vi "Main UI.vi"() -> ()   [LabVIEW 2013]
uses:
  Refactor/TypeDefs/Throttle.ctl
  Refactor/TypeDefs/Steering.ctl
  <vilib>/userdefined/High Color/IMAQdx.ctl
  Refactor/TypeDefs/PhoneIMU.ctl
  <vilib>/Utility/inputDevices.llb/joystickAcquire.vi
  PCTx Files/PCTx/PCTx.lvlib
  <vilib>/vision/driver/NI_Vision_Acquisition_Software.lvlib
  <resource>/objmgr/imaqdx.rc
  FFConstdll/FFConstDll.dll
  user32.dll
panel:
  out "Gear":i32
  in  "Tab Control":enum32{"HUD", "Stats for Nerds", "Debug Info"}(tab)
  in  "stop":bool
  out "Steering":i32(knob) scale=-32768.0..32767.0
  out "Throttle":i32(knob) scale=-32768.0..32767.0
  out "Brake":i32(slide) scale=32767.0..-32768.0
  out "Image":T1(plugin-control)
  out "Throttle Graph":cluster{dbl[], dbl[]}[](graph)
  out "Steering Graph":cluster{dbl[], dbl[]}[](graph)
  out "Raw Wheel Inputs":T2
  in  "Throttle Cluster":T3={"Neutral Signal"=512.0, "Bottom Deadzone"=707.070707070707, "Neutral Deadzone"=0.0, "Top Cutout"=971.4285714285714, "Bottom Cutout"=89.79591836734694, "Top Deadzone"=64627.90909090909, "Throttle Curve Type"=enum."Linear"} {"Top Deadzone" scale=55537.0..65537.0; "Bottom Cutout" scale=0.0..200.0; "Top Cutout" scale=800.0..1024.0; "Neutral Deadzone" scale=0.0..10000.0; "Bottom Deadzone" scale=1.0..10000.0; "Neutral Signal" scale=480.0..544.0}
  in  "Steering Cluster":T4={"Neutral Signal"=642.8571428571429, "Bottom Deadzone"=707.070707070707, "Neutral Deadzone"=0.0, "Top Cutout"=971.4285714285714, "Bottom Cutout"=89.79591836734694, "Top Deadzone"=64627.90909090909, "Throttle Curve Type"=enum."Linear"} {"Top Deadzone" scale=32768.0..65537.0; "Bottom Cutout" scale=0.0..512.0; "Top Cutout" scale=800.0..1024.0; "Neutral Deadzone" scale=0.0..10000.0; "Bottom Deadzone" scale=1.0..32767.0; "Neutral Signal" scale=420.0..700.0}
  out "Steering PPM":dbl
  out "Throttle PPM":dbl
  in  "Min Throttle":dbl=513.0
  in  "Min Reverse":dbl=511.0
  in  "CD timer":u32=250
  in  "Camera Name":T5="cam0"
  in  "Video Modes":i32(listbox)=22
  out "Start ForegroundWindow HWND":u32
  in  "nXForce":i32(slide) scale=-10000.0..10000.0
  out "SetDeviceForce HRESULT":i32
  out "Acquire HRESULT":i32
  out "Current ForegroundWindow HWND":u32
  in  "millisecond multiple":u32=50
  out "Init HRESULT":i32
  out "button info":T6
  in  "Host Port":u16=55555
  out "Source Address":u32
  out "Time Since Last Packet":u32
  out "Iteration":i32
  out "Length":i32
  out "Source Port":u16
  out "data out":string
  out "IMU Data Array":dbl[](array[numeric])
  out "output cluster":T7
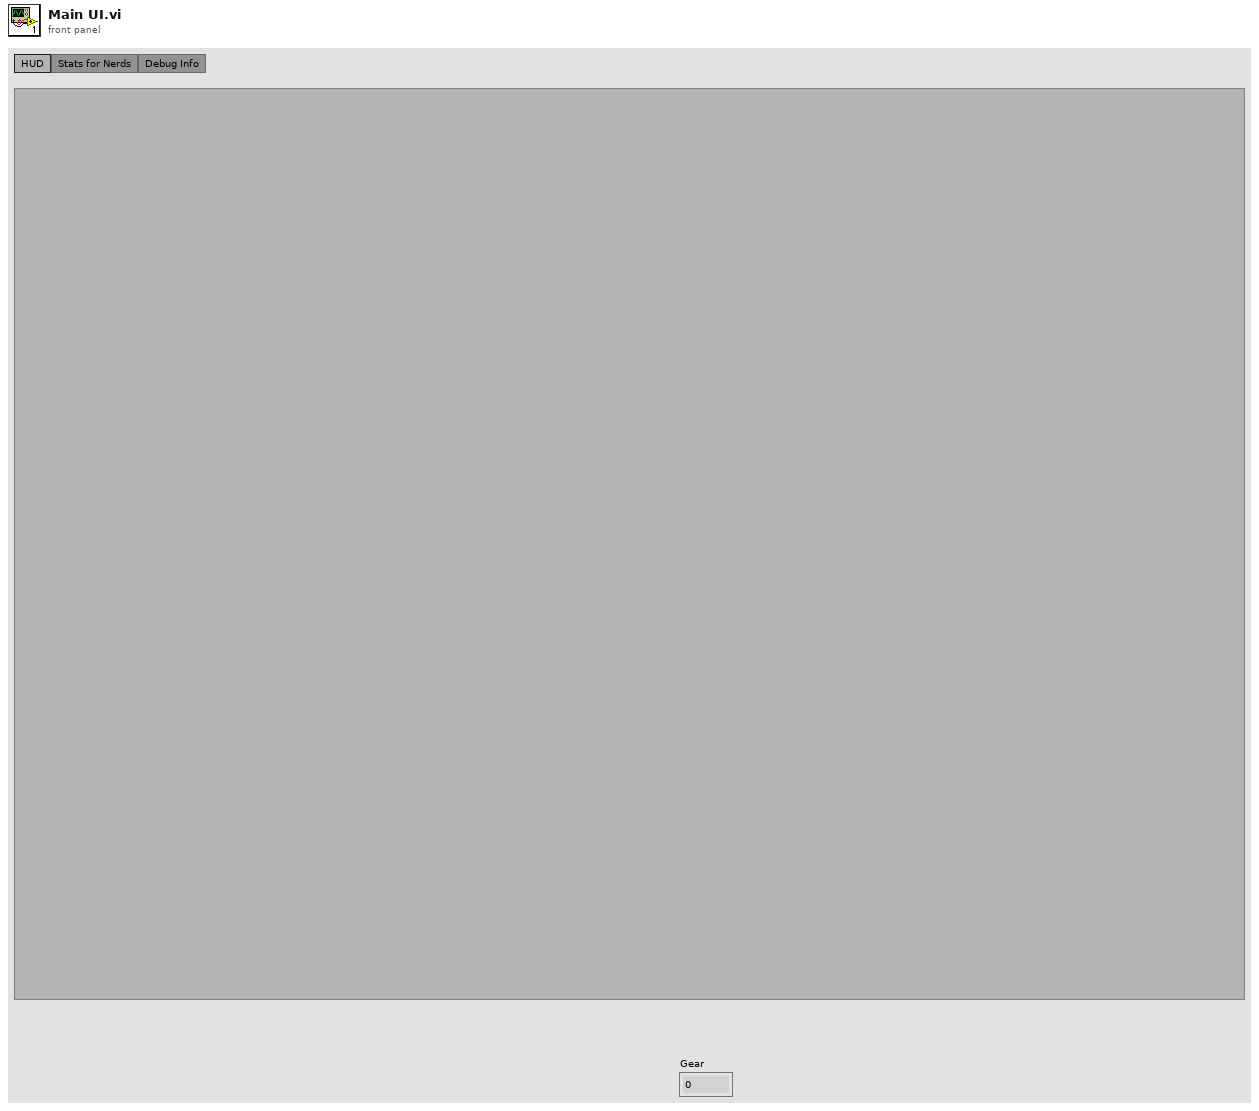
[diagram p1: front panel]
types:
  T1 = typedef "IMAQ Image.ctl" = refnum<image>
  T2 = cluster{"X axis":i32, "Y axis":i32, "Z axis":i32, "X axis rotation":i32, "Y axis rotation":i32, "Z axis rotation":i32, "U axis":i32, "V axis":i32}
  T3 = typedef "Throttle.ctl" = cluster{"Neutral Signal":dbl, "Bottom Deadzone":dbl, "Neutral Deadzone":dbl, "Top Cutout":dbl, "Bottom Cutout":dbl, "Top Deadzone":dbl, "Throttle Curve Type":enum16{"Linear", "Linear, No Deadzone", "Logarithmic", "Exponental"}}
  T4 = typedef "Steering.ctl" = cluster{"Neutral Signal":dbl, "Bottom Deadzone":dbl, "Neutral Deadzone":dbl, "Top Cutout":dbl, "Bottom Cutout":dbl, "Top Deadzone":dbl, "Throttle Curve Type":enum16{"Linear", "Linear, No Deadzone", "Logarithmic", "Exponental"}}
  T5 = typedef "IMAQdx.ctl" = refnum<k21>
  T6 = cluster{"X":bool, "Square":bool, "Circle":bool, "Triangle":bool, "Right Paddle":bool, "Left Paddle":bool, "R2":bool, "L2":bool, "Select":bool, "Start":bool, "R3":bool, "L3":bool, "Shifter +":bool, "Shifter -":bool, "Enter":bool, "Plus":bool, "Ring Clockwise":bool, "Ring CCW":bool, "Minus":bool, "GT (Center)":bool, "PS":bool, "button 22":bool, "button 23":bool, "button 24":bool, "button 25":bool, "button 26":bool, "button 27":bool, "button 28":bool, "button 29":bool, "button 30":bool, "button 31":bool, "button 32":bool}
  T7 = cluster{"Z Gyroscope":dbl, "Y Accelerometer":dbl, "X Gyroscope":dbl, "Timestamp":dbl, "Y Gyroscope":dbl, "Z Accelerometer":dbl, "GPS 5":dbl, "X Accelerometer":dbl, "X Magnetic Field":dbl, "Y Magnetic Field":dbl, "Z Magnetic Field":dbl, "GPS 1":dbl, "GPS 2":dbl, "GPS 3":dbl, "GPS 4":dbl, "GPS 6":dbl}
  T8 = typedef "PhoneIMU.ctl" = cluster{"Z Gyroscope":dbl, "Y Accelerometer":dbl, "X Gyroscope":dbl, "Timestamp":dbl, "Y Gyroscope":dbl, "Z Accelerometer":dbl, "GPS 5":dbl, "X Accelerometer":dbl, "X Magnetic Field":dbl, "Y Magnetic Field":dbl, "Z Magnetic Field":dbl, "GPS 1":dbl, "GPS 2":dbl, "GPS 3":dbl, "GPS 4":dbl, "GPS 6":dbl}
  T9 = typedef "Image Type" = u32
  T10 = cluster{"button 1":bool, "button 2":bool, "button 3":bool, "button 4":bool, "button 5":bool, "button 6":bool, "button 7":bool, "button 8":bool, "button 9":bool, "button 10":bool, "button 11":bool, "button 12":bool, "button 13":bool, "button 14":bool, "button 15":bool, "button 16":bool, "button 17":bool, "button 18":bool, "button 19":bool, "button 20":bool, "button 21":bool, "button 22":bool, "button 23":bool, "button 24":bool, "button 25":bool, "button 26":bool, "button 27":bool, "button 28":bool, "button 29":bool, "button 30":bool, "button 31":bool, "button 32":bool}
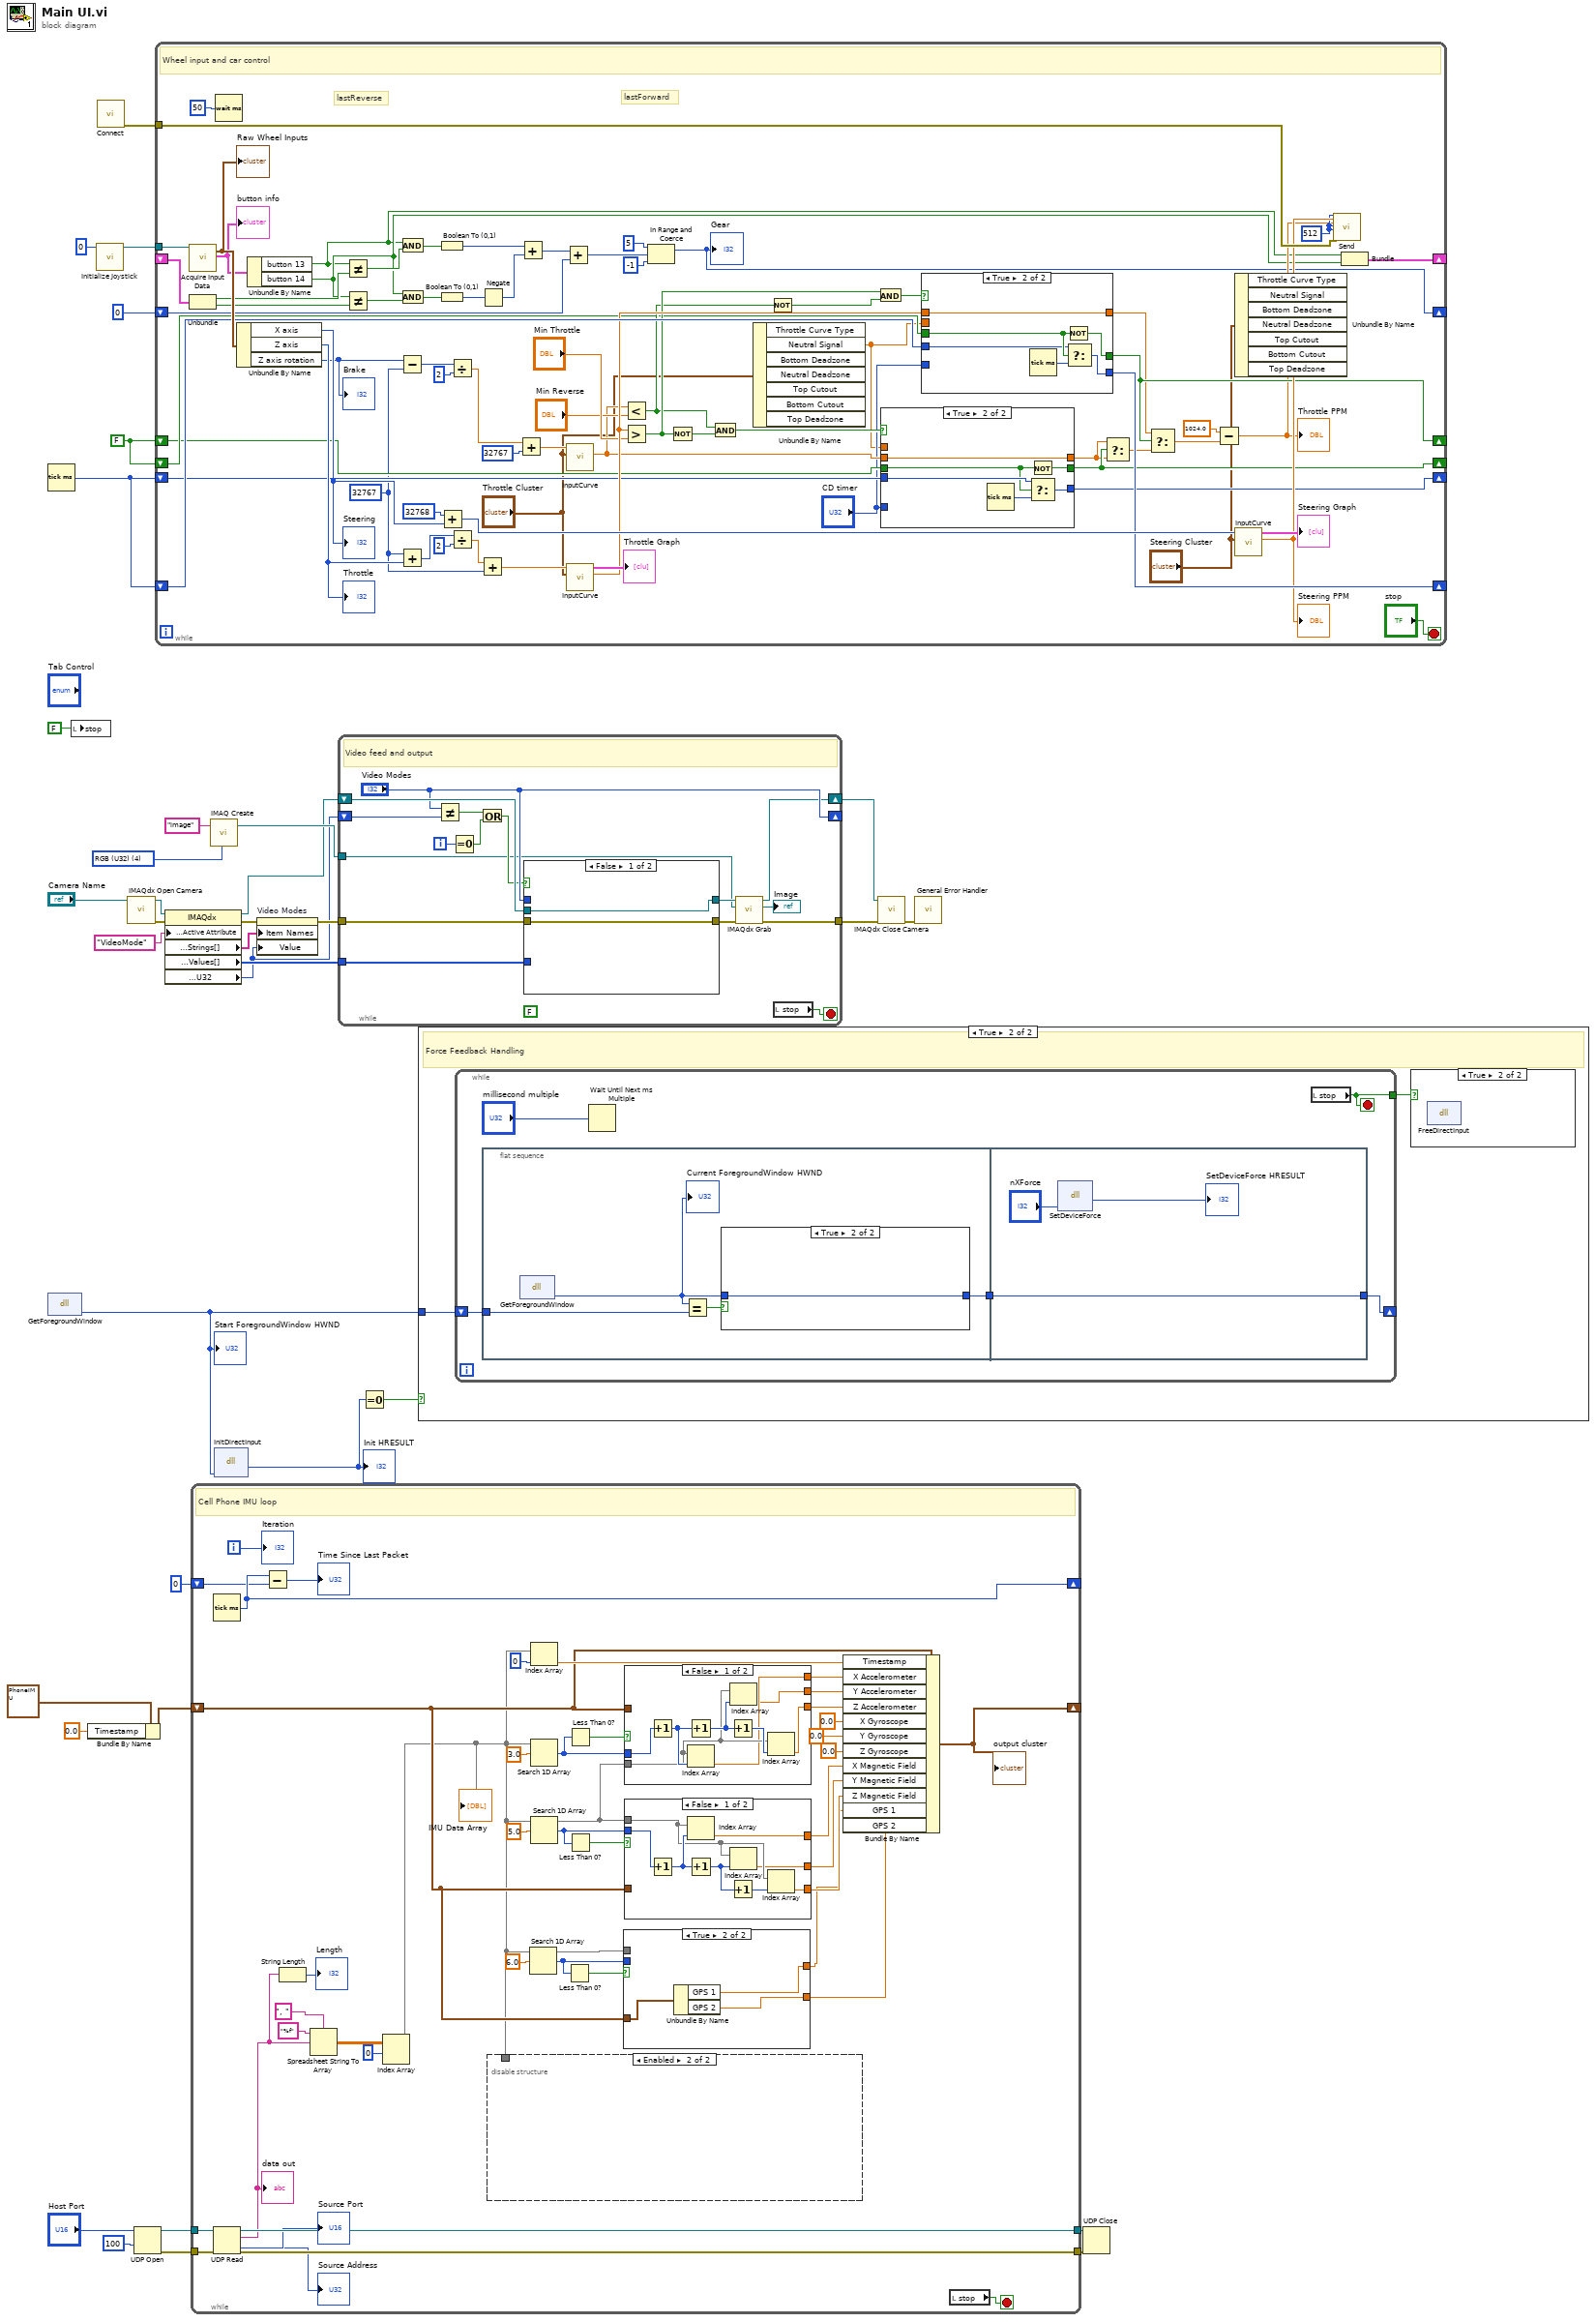
[diagram p0: block diagram]
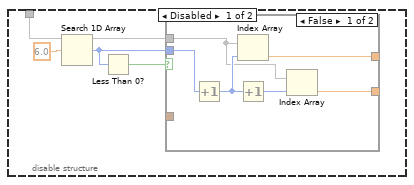
[diagram p2: hidden frame]
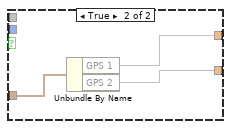
[diagram p3: hidden frame]
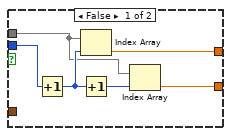
[diagram p4: hidden frame]
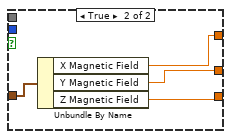
[diagram p5: hidden frame]
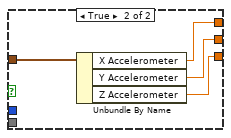
[diagram p6: hidden frame]
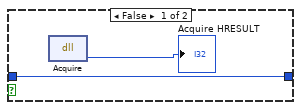
[diagram p9: hidden frame]
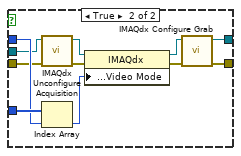
[diagram p10: hidden frame]
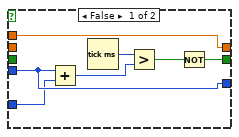
[diagram p11: hidden frame]
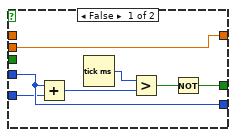
[diagram p12: hidden frame]
diagram:
  w16 = T9 4 items=["Grayscale (U8)", "Grayscale (I16)", "Grayscale (SGL)", "Complex (CSG)", "RGB (U32)", "HSL (U32)", "RGB (U64)", "Grayscale (U16)"] ("Image Type")
  w32 = FALSE
  n1 = Tick Count (ms)() -> (millisecond timer value=w33:u32)
  n2 = dll-call lib="user32.dll" fn="GetForegroundWindow"() -> ("HWND"=w13:u32)  [unwired: 3 in, 2 out]
  "Start ForegroundWindow HWND" <- w13
  n3 = local write "stop"(FALSE ("stop")) -> ()
  n4 = Bundle By Name(cluster=T8 {"Z Gyroscope"=0.0, "Y Accelerometer"=0.0, "X Gyroscope"=0.0, "Timestamp"=0.0, "Y Gyroscope"=0.0, "Z Accelerometer"=0.0, "GPS 5"=0.0, "X Accelerometer"=0.0, "X Magnetic Field"=0.0, "Y Magnetic Field"=0.0, "Z Magnetic Field"=0.0, "GPS 1"=0.0, "GPS 2"=0.0, "GPS 3"=0.0, "GPS 4"=0.0, "GPS 6"=0.0} ("input cluster"), "Timestamp"=0.0) -> (w2:T8)
  n5 = call <vilib>:"Initialize Joystick.vi"("device index"=0) -> ("device ID"=w34:refnum<k1>)  [unwired: 9 in, 1 out]
  n6 = call "Connect.vi"() -> ("error out"=w36:errorcluster)  [unwired: 10 in, 1 out]
  n7 = call <vilib>:"IMAQdx Open Camera.vi"("Session In"="Camera Name") -> ("error out"=w22:errorcluster, "Session Out"=w25:T5)  [unwired: 2 in, 7 out]
  n8 = UDP Open(9:100 ("timeout ms (25000)"), 11:"Host Port") -> (port=w6:refnum<k16>, 0:w7:errorcluster)  [unwired: 3 in, 1 out]
  n9 = while {
    tunnel: w36 -> [w106]
    tunnel: w34 -> [w105]
    shift-right: [w93] -> _
    shift-left: w33 -> [w92]
    shift-right: [w86] -> _
    shift-left: w33 -> [w87]
    shift-right: [w75] -> _
    shift-left: w32 -> [w77]
    shift-right: [w72] -> _
    shift-left: w32 -> [w78]
    shift-right: [w52] -> _
    shift-left: 0 ("device index") -> [w49]
    shift-right: [w59] -> _
    shift-left: _ -> [w58]
    stop <- "stop" stop-if-true
    w63 = 32767 ("x")
    w76 = 512
    # "lastReverse"
    # "lastForward"
    # "Wheel input and car control"
    n10 = call-poly <vilib>:"Acquire Input Data.vi"("device ID"=w105) -> ("axis info"=w104:T2, "button info"=w60:T10)  [unwired: 14 in, 3 out]
    "Raw Wheel Inputs" <- w104
    "button info" <- w60
    n11 = Unbundle(w58) -> ("button 13"=w57:bool, "button 14"=w56:bool)
    n12 = Wait (ms)(milliseconds to wait=u32 50) -> ()  [unwired: 1 out]
    n13 = Unbundle By Name(w104) -> ("X axis"=w101:i32, "Z axis"=w100:i32, "Z axis rotation"=w96:i32)
    "Steering" <- w101
    "Throttle" <- w100
    "Brake" <- w96
    n14 = Unbundle By Name(w60) -> ("button 13"=w38:bool, "button 14"=w42:bool)
    n15 = Not Equal?(x=w38, y=w57) -> (x != y?=w44:bool)
    n16 = Not Equal?(x=w42, y=w56) -> (x != y?=w43:bool)
    n17 = Subtract(x=w96, y=w63) -> (x-y=w95:i32)
    n18 = Add(x=w63, y=w100) -> (x+y=w99:i32)
    n19 = And(x=w38, y=w44) -> (x .and. y?=w46:bool)
    n20 = And(x=w42, y=w43) -> (x .and. y?=w45:bool)
    n21 = Boolean To (0,1)(Boolean=w46) -> (0, 1=w54:i16)
    n22 = Boolean To (0,1)(Boolean=w45) -> (0, 1=w55:i16)
    n23 = Add(x=32768, y=w101) -> (x+y=w102:i32)
    n24 = Divide(x=w95, y=2) -> (x/y=w70:dbl)
    n25 = Divide(x=w99, y=2) -> (x/y=w64:dbl)
    n26 = Add(x=w64, y=w63) -> (x+y=w62:dbl)
    n27 = Negate(x=w55) -> (-x=w53:i16)
    n28 = Add(x=w70, y=32767) -> (x+y=w69:dbl)
    n29 = Add(x=w54, y=w53) -> (x+y=w48:i16)
    n30 = Add(x=w48, y=w49) -> (x+y=w47:i32)
    n31 = call "InputCurve.vi"("Throttle Cluster"="Throttle Cluster", "Input"=w69) -> ("Output"=w79:dbl)  [unwired: 8 in, 1 out]
    n32 = call "InputCurve.vi"("Throttle Cluster"="Throttle Cluster", "Input"=w62) -> ("Output"=w90:dbl, "Throttle Graph"=→"Throttle Graph":cluster{dbl[], dbl[]}[])  [unwired: 8 in]
    n33 = Less?(x=w79, y="Min Reverse") -> (x < y?=w81:bool)
    n34 = Greater?(x=w90, y="Min Throttle") -> (0:w82:bool)
    n35 = In Range and Coerce(upper limit=5, x=w47, lower limit=-1) -> (coerced(x)=w52:i32)  [unwired: 1 out]
    "Gear" <- w52
    n36 = Not(x=w82) -> (.not. x?=w83:bool)
    n37 = And(x=w81, y=w83) -> (x .and. y?=w80:bool)
    n38 = Unbundle By Name("Throttle Cluster") -> ("Neutral Signal"=w40:dbl)  [unwired: 6 out]
    n39 = Not(x=w81) -> (.not. x?=w84:bool)
    n40 = And(x=w82, y=w84) -> (x .and. y?=w85:bool)
    n41 = case shown="True" w80 {
      tunnel: w87 -> [w115 w120]
      tunnel: [w115 w118] -> w86
      tunnel: [w111 w121] -> w72
      tunnel: w79 -> [_ w116]
      tunnel: w77 -> [_ w117]
      tunnel: [w110 w116] -> w37
      tunnel: w40 -> [w110 _]
      tunnel: "CD timer" -> [w109 _]
      frame False {
        n42 = Add(x=w115, y=w109) -> (x+y=w114:u32)
        n43 = Tick Count (ms)() -> (millisecond timer value=w113:u32)
        n44 = Greater?(x=w113, y=w114) -> (0:w112:bool)
        n45 = Not(x=w112) -> (.not. x?=w111:bool)
      }
      frame True {
        n46 = Tick Count (ms)() -> (millisecond timer value=w119:u32)
        n47 = Not(x=w117) -> (.not. x?=w121:bool)
        n48 = Select(t=w120, s=w117, f=w119) -> (s? t:f=w118:u32)
      }
    }
    n49 = case shown="True" w85 {
      tunnel: [w128 w130] -> w93
      tunnel: w92 -> [w128 w131]
      tunnel: w90 -> [_ w129]
      tunnel: [w124 w134] -> w75
      tunnel: w78 -> [_ w133]
      tunnel: [w123 w129] -> w74
      tunnel: w40 -> [w123 _]
      tunnel: "CD timer" -> [w122 _]
      frame False {
        n50 = Add(x=w128, y=w122) -> (x+y=w126:u32)
        n51 = Tick Count (ms)() -> (millisecond timer value=w127:u32)
        n52 = Greater?(x=w127, y=w126) -> (0:w125:bool)
        n53 = Not(x=w125) -> (.not. x?=w124:bool)
      }
      frame True {
        n54 = Tick Count (ms)() -> (millisecond timer value=w132:u32)
        n55 = Not(x=w133) -> (.not. x?=w134:bool)
        n56 = Select(t=w131, s=w133, f=w132) -> (s? t:f=w130:u32)
      }
    }
    n57 = Select(t=w37, s=w72, f=w37) -> (s? t:f=w73:dbl)
    n58 = Select(t=w74, s=w75, f=w73) -> (s? t:f=w67:dbl)
    n59 = Subtract(x=1024.0, y=w67) -> (x-y=w68:dbl)
    "Throttle PPM" <- w68
    n60 = Unbundle By Name("Steering Cluster") -> ()  [unwired: 7 out]
    n61 = call "InputCurve.vi"("Throttle Cluster"="Steering Cluster", "Input"=w102) -> ("Output"=w91:dbl, "Throttle Graph"=→"Steering Graph":cluster{dbl[], dbl[]}[])  [unwired: 8 in]
    "Steering PPM" <- w91
    n62 = call "Send.vi"("Ch1"=w76, "Ch2"=w91, "Ch3"=w68, "Ch4"=w76, "Ch5"=w76, "error in (no error)"=w106) -> ()  [unwired: 20 in, 2 out]
    n63 = Bundle("button 13"=w38, "button 14"=w42) -> (w59:cluster{"button 13":bool, "button 14":bool})  [unwired: 1 in]
  }
  n64 = property class="IMAQdx"(reference=w25, error in=w22, "Camera Attributes:Active Attribute"="VideoMode" ("ActiveAttribute")) -> (reference out=w20:T5, error out=w21:errorcluster, "Camera Attributes:Enum:Strings[]"=w18:string[], "Camera Attributes:Enum:Values[]"=w23:u32[], "Camera Attributes:Value:U32"=w17:u32)
  n65 = while {
    tunnel: w6 -> [w176]
    tunnel: w7 -> [w175]
    tunnel: [w174] -> w9
    tunnel: [w173] -> w8
    shift-right: [w168] -> _
    shift-left: u32 0 ("millisecond timer value") -> [w167]
    shift-right: [w145] -> _
    shift-left: w2 -> [w138]
    i -> [w169]
    stop <- w165 stop-if-true
    # "Cell Phone IMU loop"
    n66 = Tick Count (ms)() -> (millisecond timer value=w168:u32)
    n67 = UDP Read(connection ID=w176, 8:w175) -> (data out=w164:string, error out=w174:errorcluster, 3:w173:refnum<k16>, 4:→"Source Port":u16, 6:→"Source Address":u32)  [unwired: 2 in]
    "data out" <- w164
    n68 = Subtract(x=w168, y=w167) -> (x-y=→"Time Since Last Packet":u32)
    n69 = String Length(string=w164) -> (length=→"Length":i32)
    n70 = Spreadsheet String To Array(delimiter (Tab)=", ", format string="%f", spreadsheet string=w164) -> (array=w161:dbl[][])  [unwired: 1 in]
    n71 = Index Array(array=w161, index (row)=0 ("index")) -> (element=w135:dbl[])  [unwired: 1 in]
    "IMU Data Array" <- w135
    n72 = disable-structure shown="Enabled" {
      disable-tunnel: w135 -> [w180 _]
      frame Disabled {
        n73 = Search 1D Array(element=6.0) -> (index of element=w178:i32)  [unwired: 2 in]
        n74 = Less Than 0?(x=w178) -> (x < 0?=w177:bool)
        n75 = case shown="False" w177 {
          tunnel: w178 -> [w186 _]
          tunnel: w180 -> [w181 _]
          tunnel: [w183 w189] -> _
          tunnel: [w182 w188] -> _
          tunnel: _ -> [_ w187]
          frame False {
            n76 = Increment(x=w186) -> (x+1=w184:i32)
            n77 = Index Array(array=w181, index=w184) -> (element=w183:dbl)
            n78 = Increment(x=w184) -> (x+1=w185:i32)
            n79 = Index Array(array=w181, index=w185) -> (element=w182:dbl)
          }
          frame True {
            n80 = Unbundle By Name(w187) -> ("GPS 1"=w189, "GPS 2"=w188)
          }
        }
      }
      frame Enabled {
      }
    }
    n81 = Search 1D Array(1D array=w135, element=6.0) -> (index of element=w139:i32)  [unwired: 1 in]
    n82 = Index Array(array=w135, index=0) -> (element=w146:dbl)
    n83 = Search 1D Array(1D array=w135, element=3.0) -> (index of element=w156:i32)  [unwired: 1 in]
    n84 = Search 1D Array(1D array=w135, element=5.0) -> (index of element=w147:i32)  [unwired: 1 in]
    n85 = Less Than 0?(x=w139) -> (x < 0?=w140:bool)
    n86 = Less Than 0?(x=w156) -> (x < 0?=w157:bool)
    n87 = Less Than 0?(x=w147) -> (x < 0?=w151:bool)
    n88 = case shown="True" w140 {
      tunnel: w139 -> [w195 _]
      tunnel: w135 -> [w190 _]
      tunnel: [w192 w198] -> w137
      tunnel: [w191 w197] -> w136
      tunnel: w138 -> [_ w196]
      frame False {
        n89 = Increment(x=w195) -> (x+1=w193:i32)
        n90 = Index Array(array=w190, index=w193) -> (element=w192:dbl)
        n91 = Increment(x=w193) -> (x+1=w194:i32)
        n92 = Index Array(array=w190, index=w194) -> (element=w191:dbl)
      }
      frame True {
        n93 = Unbundle By Name(w196) -> ("GPS 1"=w198:dbl, "GPS 2"=w197:dbl)
      }
    }
    n94 = case shown="False" w157 {
      tunnel: w156 -> [w218 _]
      tunnel: w135 -> [w214 _]
      tunnel: [w213 w221] -> w155
      tunnel: [w212 w220] -> w154
      tunnel: [w211 w219] -> w153
      tunnel: w138 -> [_ w222]
      frame False {
        n95 = Increment(x=w218) -> (x+1=w215:i32)
        n96 = Increment(x=w215) -> (x+1=w216:i32)
        n97 = Index Array(array=w214, index=w215) -> (element=w213:dbl)
        n98 = Increment(x=w216) -> (x+1=w217:i32)
        n99 = Index Array(array=w214, index=w216) -> (element=w212:dbl)
        n100 = Index Array(array=w214, index=w217) -> (element=w211:dbl)
      }
      frame True {
        n101 = Unbundle By Name(w222) -> ("X Accelerometer"=w221:dbl, "Y Accelerometer"=w220:dbl, "Z Accelerometer"=w219:dbl)
      }
    }
    n102 = case shown="False" w151 {
      tunnel: w147 -> [w206 _]
      tunnel: w135 -> [w202 _]
      tunnel: [w201 w210] -> w150
      tunnel: [w200 w209] -> w149
      tunnel: [w199 w208] -> w148
      tunnel: w138 -> [_ w207]
      frame False {
        n103 = Increment(x=w206) -> (x+1=w203:i32)
        n104 = Index Array(array=w202, index=w203) -> (element=w201:dbl)
        n105 = Increment(x=w203) -> (x+1=w204:i32)
        n106 = Increment(x=w204) -> (x+1=w205:i32)
        n107 = Index Array(array=w202, index=w204) -> (element=w200:dbl)
        n108 = Index Array(array=w202, index=w205) -> (element=w199:dbl)
      }
      frame True {
        n109 = Unbundle By Name(w207) -> ("X Magnetic Field"=w210:dbl, "Y Magnetic Field"=w209:dbl, "Z Magnetic Field"=w208:dbl)
      }
    }
    n110 = Bundle By Name(cluster=w138, "Timestamp"=w146, "X Accelerometer"=w155, "Y Accelerometer"=w154, "Z Accelerometer"=w153, "X Gyroscope"=0.0, "Y Gyroscope"=0.0, "Z Gyroscope"=0.0, "X Magnetic Field"=w150, "Y Magnetic Field"=w149, "Z Magnetic Field"=w148, "GPS 1"=w137, "GPS 2"=w136) -> (w145:T8)
    "output cluster" <- w145
    n111 = local read "stop"() -> (w165:bool)
    "Iteration" <- w169
  }
  n112 = call "IMAQ Create"("Image Name"="image", "Image Type"=w16) -> ("New Image"=w28:T1)  [unwired: 2 in, 2 out]
  n113 = dll-call lib="E:/Documents and Files/LabVIEW Projects/KURT Teleop/Winter '14 Force Feedback Experiment/FFConstdll/FFConstDll.dll" fn="InitDirectInput"("hDlg"=w13) -> ("HRESULT"=w12:u32)  [unwired: 4 in, 2 out]
  "Init HRESULT" <- w12
  n114 = property on="Video Modes" class="LstBox (strict)"(error in=w21, "Item Names"=w18, "Value"=w17) -> (error out=w19:errorcluster)  [unwired: 1 in, 1 out]
  n115 = while {
    tunnel: w23 -> [w236]
    shift-left: w17 -> [w235]
    shift-right: ["Video Modes"] -> _
    tunnel: w28 -> [w225]
    tunnel: w19 -> [w237]
    tunnel: [w227] -> w30
    shift-right: [w228] -> w27
    shift-left: w20 -> [w238]
    i -> [w224]
    stop <- w223 stop-if-true
    (unwired) FALSE
    # "Video feed and output"
    n116 = Not Equal?(x="Video Modes", y=w235) -> (x != y?=w232:bool)
    n117 = Equal To 0?(x=w224) -> (x = 0?=w231:bool)
    n118 = Or(x=w232, y=w231) -> (x .or. y?=w233:bool)
    n119 = case shown="False" w233 {
      tunnel: w238 -> [w240 w249]
      tunnel: w237 -> [w239 w248]
      tunnel: [w240 w245] -> w229
      tunnel: [w239 w246] -> w230
      tunnel: w236 -> [_ w251]
      tunnel: "Video Modes" -> [_ w250]
      frame False {
      }
      frame True {
        n120 = call <vilib>:"IMAQdx Unconfigure Acquisition.vi"("error in"=w248, "Session In"=w249) -> ("error out"=w242:errorcluster, "Session Out"=w247:T5)  [unwired: 8 out]
        n121 = Index Array(array=w251, index=w250) -> (element=w241:u32)
        n122 = property class="IMAQdx"(reference=w247, error in=w242, "Acquisition Attributes:Video Mode"=w241) -> (reference out=w244:T5, error out=w243:errorcluster)
        n123 = call <vilib>:"IMAQdx Configure Grab.vi"("error in"=w243, "Session In"=w244) -> ("error out"=w246:errorcluster, "Session Out"=w245:T5)  [unwired: 1 in, 7 out]
      }
    }
    n124 = call <vilib>:"IMAQdx Grab.vi"("error in"=w230, "Image In"=w225, "Session In"=w229) -> ("error out"=w227:errorcluster, "Image Out"=→"Image":T1, "Session Out"=w228:T5)  [unwired: 1 in, 5 out]
    n125 = local read "stop"() -> (w223:bool)
  }
  n126 = Equal To 0?(x=w12) -> (x = 0?=w14:bool)
  n127 = case shown="True" w14 {
    tunnel: w13 -> [_ w252]
    frame False {
    }
    frame True {
      # "Force Feedback Handling"
      n128 = while {
        tunnel: [w254] -> w253
        shift-right: [w258] -> _
        shift-left: w252 -> [w256]
        stop <- w254 stop-if-true
        n129 = flat-sequence {
          tunnel: w256 -> [w262]
          tunnel: [w259] -> w257
          tunnel: [w266] -> w258
          tunnel: w257 -> [w266]
          frame #0 {
            n130 = dll-call lib="user32.dll" fn="GetForegroundWindow"() -> ("HWND"=w260:u32)  [unwired: 3 in, 2 out]
            "Current ForegroundWindow HWND" <- w260
            n131 = Equal?(x=w260, y=w262) -> (x = y?=w261:bool)
            n132 = case shown="True" w261 {
              tunnel: w260 -> [w263 w265]
              tunnel: [w263 w265] -> w259
              frame False {
                n133 = dll-call lib="E:/Documents and Files/LabVIEW Projects/KURT Teleop/Winter '14 Force Feedback Experiment/FFConstdll/FFConstDll.dll" fn="Acquire"() -> ("HRESULT"=→"Acquire HRESULT":i32)  [unwired: 3 in, 2 out]
              }
              frame True {
              }
            }
          }
          frame #1 {
            n134 = dll-call lib="E:/Documents and Files/LabVIEW Projects/KURT Teleop/Winter '14 Force Feedback Experiment/FFConstdll/FFConstDll.dll" fn="SetDeviceForce"("nXForce"="nXForce") -> ("HRESULT"=→"SetDeviceForce HRESULT":i32)  [unwired: 4 in, 2 out]
          }
        }
        n135 = Wait Until Next ms Multiple(millisecond multiple="millisecond multiple") -> ()  [unwired: 1 out]
        n136 = local read "stop"() -> (w254:bool)
      }
      n137 = case shown="True" w253 {
        frame False {
        }
        frame True {
          n138 = dll-call lib="E:/Documents and Files/LabVIEW Projects/KURT Teleop/Winter '14 Force Feedback Experiment/FFConstdll/FFConstDll.dll" fn="FreeDirectInput"() -> ()  [unwired: 4 in, 2 out]
        }
      }
    }
  }
  n139 = call <vilib>:"IMAQdx Close Camera.vi"("error in"=w30, "Session In"=w27) -> ("error out"=w31:errorcluster)  [unwired: 9 out]
  n140 = call <vilib>:"General Error Handler.vi"("error in (no error)"=w31) -> ()  [unwired: 1 in, 14 out]
  n141 = UDP Close(connection ID=w8, 8:w9) -> ()  [unwired: 2 out]
